vi "초음파센서.vi"() -> ()   [LabVIEW 2018]
uses:
  <vilib>/DAQmx/read.llb/DAQmx Read (Counter DBL 1Chan 1Samp).vi
  <vilib>/DAQmx/write.llb/DAQmx Write (Digital Bool 1Line 1Point).vi
  <vilib>/DAQmx/create/channels.llb/DAQmx Create Channel (DO-Digital Output).vi
  <vilib>/DAQmx/create/channels.llb/DAQmx Create Channel (CI-Pulse Width).vi
  <vilib>/DAQmx/miscellaneous.llb/DAQmx Fill In Error Info.vi
panel:
  out "거리(cm)":dbl(slide) scale=0.0..50.0
  in  "정지 버튼":bool
  in  "수신부 카운터":tag caption="카운터"
  in  "lines":tag caption="라인"
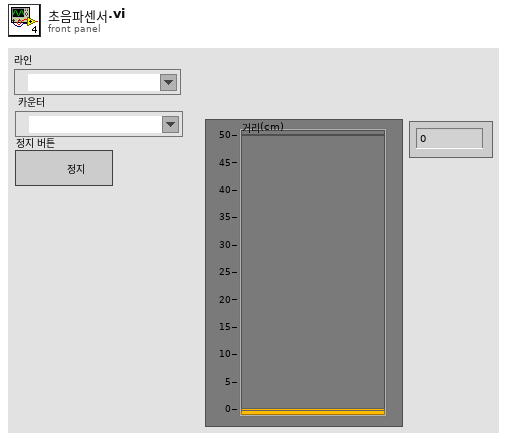
[diagram p1: front panel]
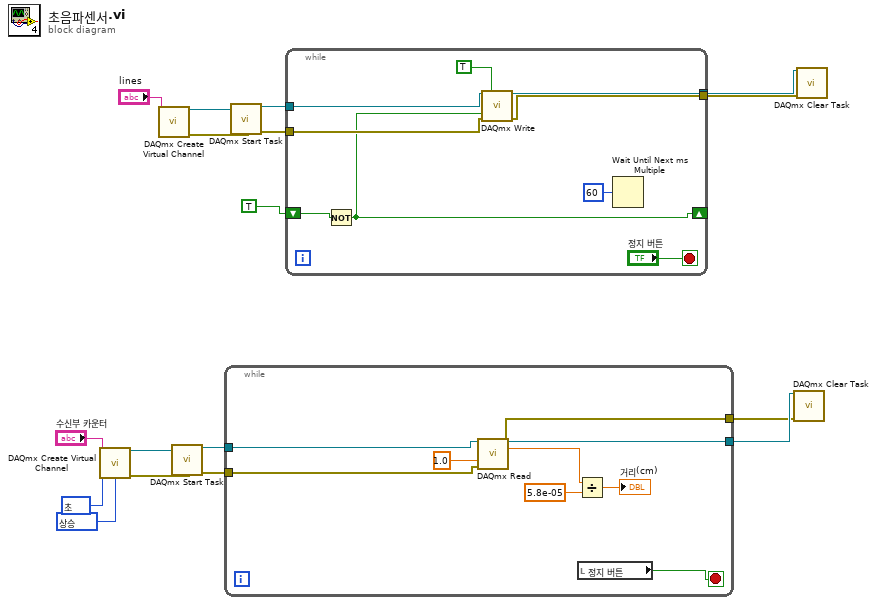
[diagram p0: block diagram]
diagram:
  w10 = 10280 items=["상승"=10280, "하강"=10171] ("starting edge")
  w11 = 10364 items=["초"=10364, "Tick"=10304, "사용자 스케일로부터"=10065] ("units")
  n1 = call-poly <vilib>:"DAQmx Create Virtual Channel.vi"("counter"="수신부 카운터", "units"=w11, "starting edge"=w10) -> ("task out"=w13:refnum<k21>, "error out"=w14:errorcluster)  [unwired: 11 in]
  n2 = call-poly <vilib>:"DAQmx Create Virtual Channel.vi"("lines"="lines") -> ("task out"=w16:refnum<k21>, "error out"=w15:errorcluster)  [unwired: 13 in]
  n3 = call <vilib>:"DAQmx Start Task.vi"("task/channels in"=w13, "error in"=w14) -> ("task out"=w4:refnum<k21>, "error out"=w3:errorcluster)  [unwired: 12 in]
  n4 = while {
    tunnel: w4 -> [w25]
    tunnel: w3 -> [w23]
    tunnel: [w22] -> w2
    tunnel: [w21] -> w1
    stop <- w26 stop-if-true
    n5 = call-poly <vilib>:"DAQmx Read.vi"("task/channels in"=w25, "timeout"=1.0, "error in"=w23) -> ("task out"=w22:refnum<k21>, "data"=w20:dbl, "error out"=w21:errorcluster)  [unwired: 10 in]
    n6 = Divide(x=w20, y=5.8e-05) -> (x/y=→"거리(cm)":dbl)
    n7 = local read "정지 버튼"() -> (w26:bool)
  }
  n8 = call <vilib>:"DAQmx Start Task.vi"("task/channels in"=w16, "error in"=w15) -> ("task out"=w9:refnum<k21>, "error out"=w8:errorcluster)  [unwired: 12 in]
  n9 = while {
    tunnel: w9 -> [w35]
    tunnel: w8 -> [w34]
    tunnel: [w33] -> w7
    tunnel: [w32] -> w6
    shift-right: [w29] -> _
    shift-left: TRUE -> [w30]
    stop <- "정지 버튼" stop-if-true
    n10 = Not(x=w30) -> (.not. x?=w29:bool)
    n11 = call-poly <vilib>:"DAQmx Write.vi"("task/channels in"=w35, "auto start"=TRUE, "data"=w29, "error in"=w34) -> ("task out"=w33:refnum<k21>, "error out"=w32:errorcluster)  [unwired: 9 in, 1 out]
    n12 = Wait Until Next ms Multiple(millisecond multiple=u32 60 ("ms 배수")) -> ()  [unwired: 1 out]
  }
  n13 = call <vilib>:"DAQmx Clear Task.vi"("task in"=w2, "error in"=w1) -> ()  [unwired: 13 in, 1 out]
  n14 = call <vilib>:"DAQmx Clear Task.vi"("task in"=w7, "error in"=w6) -> ()  [unwired: 13 in, 1 out]
